vi "Yellow 1 to 2.vi"   [LabVIEW 2019]
uses:
  Global Var.vi
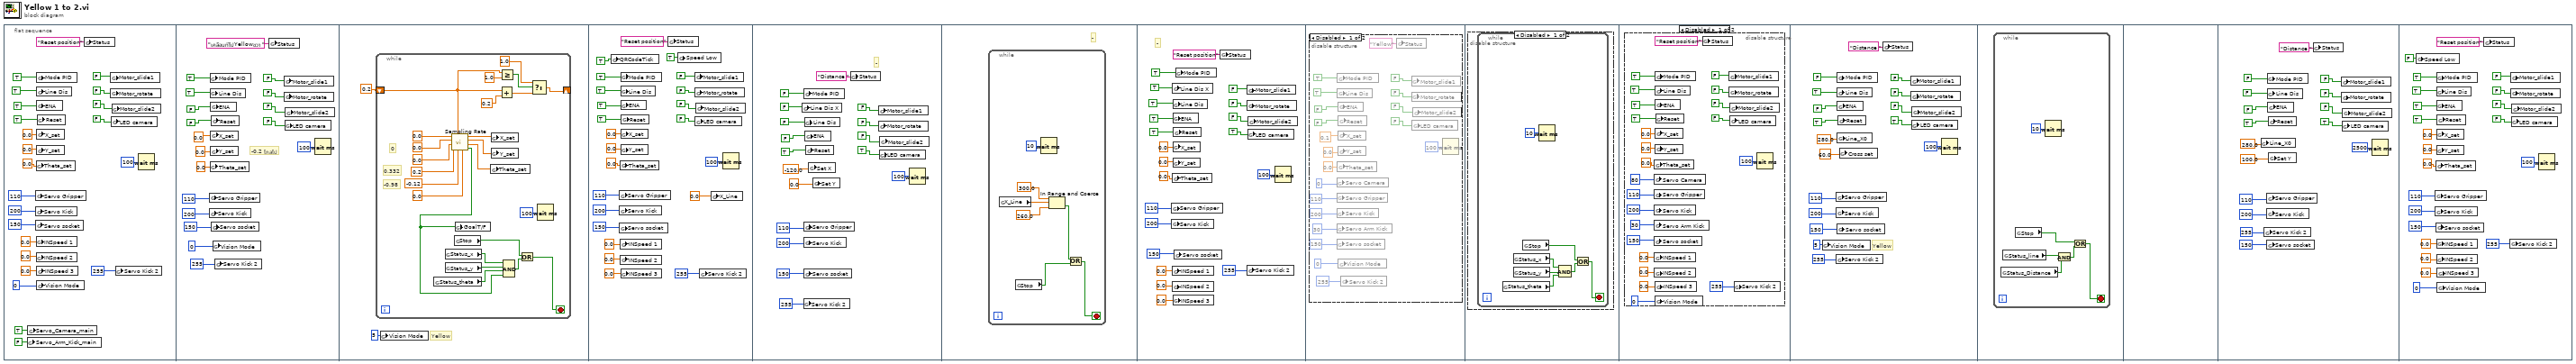
[diagram p0: block diagram]
diagram:
  n1 = flat-sequence {
    frame #0 {
      n2 = global write "Global Var.vi" "Servo_Arm_Kick_main"(FALSE ("Mode PID")) -> ()
      n3 = global write "Global Var.vi" "Servo_Camera_main"(TRUE ("Mode PID")) -> ()
      n4 = global write "Global Var.vi" "Servo Gripper"(u8 110 ("Servo Camera")) -> ()
      n5 = global write "Global Var.vi" "Servo Kick"(u8 200 ("Servo Camera")) -> ()
      n6 = global write "Global Var.vi" "Servo socket"(u8 150 ("Servo Camera")) -> ()
      n7 = global write "Global Var.vi" "Theta_set"(0.0 ("Theta_set")) -> ()
      n8 = global write "Global Var.vi" "INSpeed 1"(0.0 ("X_set")) -> ()
      n9 = global write "Global Var.vi" "INSpeed 2"(0.0 ("Y_set")) -> ()
      n10 = global write "Global Var.vi" "Mode PID"(TRUE ("Mode PID")) -> ()
      n11 = global write "Global Var.vi" "Line Dis"(TRUE ("Mode PID")) -> ()
      n12 = global write "Global Var.vi" "ENA"(TRUE ("ENA")) -> ()
      n13 = global write "Global Var.vi" "X_set"(0.0 ("X_set")) -> ()
      n14 = global write "Global Var.vi" "Y_set"(0.0 ("Y_set")) -> ()
      n15 = global write "Global Var.vi" "INSpeed 3"(0.0 ("Theta_set")) -> ()
      n16 = global write "Global Var.vi" "Vision Mode"(i16 0 ("Vision Mode")) -> ()
      n17 = global write "Global Var.vi" "Reset"(TRUE ("ENA")) -> ()
      n18 = global write "Global Var.vi" "Status"("Reset position" ("Status")) -> ()
      n19 = global write "Global Var.vi" "Motor_slide1"(FALSE ("Mode PID")) -> ()
      n20 = global write "Global Var.vi" "Motor_rotate"(FALSE ("ENA")) -> ()
      n21 = global write "Global Var.vi" "LED camera"(FALSE ("LED camera")) -> ()
      n22 = global write "Global Var.vi" "Motor_slide2"(FALSE ("ENA")) -> ()
      n23 = global write "Global Var.vi" "Servo Kick 2"(u8 255 ("Servo Camera")) -> ()
      n24 = Wait (ms)(milliseconds to wait=u32 100) -> ()  [unwired: 1 out]
    }
    frame #1 {
      # "-0.2 ไกลไป"
      n25 = global write "Global Var.vi" "Servo Gripper"(u8 110 ("Servo Camera")) -> ()
      n26 = global write "Global Var.vi" "Servo Kick"(u8 200 ("Servo Camera")) -> ()
      n27 = global write "Global Var.vi" "Mode PID"(TRUE ("Mode PID")) -> ()
      n28 = global write "Global Var.vi" "Line Dis"(TRUE ("Mode PID")) -> ()
      n29 = global write "Global Var.vi" "Theta_set"(0.0 ("Theta_set")) -> ()
      n30 = global write "Global Var.vi" "ENA"(FALSE ("ENA")) -> ()
      n31 = global write "Global Var.vi" "X_set"(0.0 ("X_set")) -> ()
      n32 = global write "Global Var.vi" "Y_set"(0.0 ("Y_set")) -> ()
      n33 = global write "Global Var.vi" "Reset"(FALSE ("ENA")) -> ()
      n34 = global write "Global Var.vi" "Servo socket"(u8 150 ("Servo Camera")) -> ()
      n35 = global write "Global Var.vi" "Vision Mode"(i16 0 ("Vision Mode")) -> ()
      n36 = global write "Global Var.vi" "Servo Kick 2"(u8 255 ("Servo Camera")) -> ()
      n37 = global write "Global Var.vi" "Status"("เคลื่อนที่ไปYellowขวา " ("Status")) -> ()
      n38 = global write "Global Var.vi" "Motor_slide1"(FALSE ("Mode PID")) -> ()
      n39 = global write "Global Var.vi" "Motor_rotate"(FALSE ("ENA")) -> ()
      n40 = global write "Global Var.vi" "LED camera"(FALSE ("LED camera")) -> ()
      n41 = global write "Global Var.vi" "Motor_slide2"(FALSE ("ENA")) -> ()
      n42 = Wait (ms)(milliseconds to wait=u32 100) -> ()  [unwired: 1 out]
    }
    frame #2 {
      # "Yellow"
      n43 = while {
        shift-right: [w46] -> _
        shift-left: 0.2 -> [w44]
        stop <- w63 stop-if-true
        # "-0.98"
        # "0"
        # "0.332"
        n44 = global read "Global Var.vi" "Status_theta"() -> (w65:bool)
        n45 = global read "Global Var.vi" "Status_x"() -> (w66:bool)
        n46 = global read "Global Var.vi" "Status_y"() -> (w67:bool)
        n47 = call "Sampling Rate.vi"("input a1"=0.0, "input y1"=-0.12, "T(0-1)"=w44, "input x1"=0.2, "input a0"=0.0, "input y0"=0.0, "input x0"=0.0) -> ("GoalT/F"=w51:bool, "a_output"=w58:dbl, "y_output"=w59:dbl, "x_output"=w60:dbl)  [unwired: 1 in]
        n48 = global read "Global Var.vi" "Stop"() -> (w61:bool)
        n49 = global write "Global Var.vi" "GoalT/F"(w51) -> ()
        n50 = global write "Global Var.vi" "Theta_set"(w58) -> ()
        n51 = global write "Global Var.vi" "X_set"(w60) -> ()
        n52 = global write "Global Var.vi" "Y_set"(w59) -> ()
        n53 = Add(x=w44, y=0.2) -> (x+y=w49:dbl)
        n54 = Greater Or Equal?(x=w44, y=1.0) -> (x >= y?=w48:bool)
        n55 = Compound Arithmetic op=AND(w66, w67, w65, w51) -> (w62:bool)
        n56 = Or(x=w61, y=w62) -> (x .or. y?=w63:bool)
        n57 = Select(t=1.0, s=w48, f=w49) -> (s? t:f=w46:dbl)
        n58 = Wait (ms)(milliseconds to wait=u32 100) -> ()  [unwired: 1 out]
      }
      n59 = global write "Global Var.vi" "Vision Mode"(i16 5 ("Vision Mode")) -> ()
    }
    frame #3 {
      n60 = global write "Global Var.vi" "QRCodeTick"(TRUE ("ENA")) -> ()
      n61 = global write "Global Var.vi" "Servo Gripper"(u8 110 ("Servo Camera")) -> ()
      n62 = global write "Global Var.vi" "Servo Kick"(u8 200 ("Servo Camera")) -> ()
      n63 = global write "Global Var.vi" "Servo socket"(u8 150 ("Servo Camera")) -> ()
      n64 = global write "Global Var.vi" "Theta_set"(0.0 ("Theta_set")) -> ()
      n65 = global write "Global Var.vi" "INSpeed 1"(0.0 ("X_set")) -> ()
      n66 = global write "Global Var.vi" "INSpeed 2"(0.0 ("Y_set")) -> ()
      n67 = global write "Global Var.vi" "Mode PID"(TRUE ("Mode PID")) -> ()
      n68 = global write "Global Var.vi" "Line Dis"(TRUE ("Mode PID")) -> ()
      n69 = global write "Global Var.vi" "ENA"(TRUE ("ENA")) -> ()
      n70 = global write "Global Var.vi" "X_set"(0.0 ("X_set")) -> ()
      n71 = global write "Global Var.vi" "Y_set"(0.0 ("Y_set")) -> ()
      n72 = global write "Global Var.vi" "INSpeed 3"(0.0 ("Theta_set")) -> ()
      n73 = global write "Global Var.vi" "Reset"(TRUE ("ENA")) -> ()
      n74 = global write "Global Var.vi" "Status"("Reset position" ("Status")) -> ()
      n75 = global write "Global Var.vi" "Speed Low"(TRUE ("ENA")) -> ()
      n76 = global write "Global Var.vi" "Motor_slide1"(FALSE ("Mode PID")) -> ()
      n77 = global write "Global Var.vi" "Motor_rotate"(FALSE ("ENA")) -> ()
      n78 = global write "Global Var.vi" "LED camera"(FALSE ("LED camera")) -> ()
      n79 = global write "Global Var.vi" "Motor_slide2"(FALSE ("ENA")) -> ()
      n80 = global write "Global Var.vi" "Servo Kick 2"(u8 255 ("Servo Camera")) -> ()
      n81 = global write "Global Var.vi" "X_Line"(0.0 ("X_set")) -> ()
      n82 = Wait (ms)(milliseconds to wait=u32 100) -> ()  [unwired: 1 out]
    }
    frame #4 {
      # "-"
      n83 = global write "Global Var.vi" "Line Dis X"(FALSE ("Mode PID")) -> ()
      n84 = global write "Global Var.vi" "Servo Kick 2"(u8 255 ("Servo Camera")) -> ()
      n85 = global write "Global Var.vi" "Mode PID"(FALSE ("Mode PID")) -> ()
      n86 = global write "Global Var.vi" "Servo Gripper"(u8 110 ("Servo Camera")) -> ()
      n87 = global write "Global Var.vi" "Servo Kick"(u8 200 ("Servo Camera")) -> ()
      n88 = global write "Global Var.vi" "Servo socket"(u8 150 ("Servo Camera")) -> ()
      n89 = global write "Global Var.vi" "Line Dis"(FALSE ("Mode PID")) -> ()
      n90 = global write "Global Var.vi" "ENA"(FALSE ("ENA")) -> ()
      n91 = global write "Global Var.vi" "Reset"(TRUE ("ENA")) -> ()
      n92 = global write "Global Var.vi" "Set X"(-120.0 ("Y_set")) -> ()
      n93 = global write "Global Var.vi" "Set Y"(0.0 ("Y_set")) -> ()
      n94 = global write "Global Var.vi" "Status"("Distance " ("Status")) -> ()
      n95 = global write "Global Var.vi" "Motor_slide1"(FALSE ("Mode PID")) -> ()
      n96 = global write "Global Var.vi" "Motor_rotate"(FALSE ("ENA")) -> ()
      n97 = global write "Global Var.vi" "LED camera"(TRUE ("LED camera")) -> ()
      n98 = global write "Global Var.vi" "Motor_slide2"(FALSE ("ENA")) -> ()
      n99 = Wait (ms)(milliseconds to wait=u32 100) -> ()  [unwired: 1 out]
    }
    frame #5 {
      # "-"
      n100 = while {
        stop <- w113 stop-if-true
        n101 = global read "Global Var.vi" "X_Line"() -> (w111:dbl)
        n102 = global read "Global Var.vi" "Stop"() -> (w112:bool)
        n103 = Wait (ms)(milliseconds to wait=u32 10) -> ()  [unwired: 1 out]
        n104 = In Range and Coerce(upper limit=300.0, x=w111, lower limit=260.0) -> (In Range?=w108:bool)  [unwired: 1 out]
        n105 = Or(x=w108, y=w112) -> (x .or. y?=w113:bool)
      }
    }
    frame #6 {
      # "-"
      n106 = global write "Global Var.vi" "Servo Gripper"(u8 110 ("Servo Camera")) -> ()
      n107 = global write "Global Var.vi" "Servo Kick"(u8 200 ("Servo Camera")) -> ()
      n108 = global write "Global Var.vi" "Line Dis X"(TRUE ("Mode PID")) -> ()
      n109 = global write "Global Var.vi" "Theta_set"(0.0 ("Theta_set")) -> ()
      n110 = global write "Global Var.vi" "INSpeed 1"(0.0 ("X_set")) -> ()
      n111 = global write "Global Var.vi" "INSpeed 2"(0.0 ("Y_set")) -> ()
      n112 = global write "Global Var.vi" "Line Dis"(TRUE ("Mode PID")) -> ()
      n113 = global write "Global Var.vi" "ENA"(TRUE ("ENA")) -> ()
      n114 = global write "Global Var.vi" "X_set"(0.0 ("X_set")) -> ()
      n115 = global write "Global Var.vi" "Y_set"(0.0 ("Y_set")) -> ()
      n116 = global write "Global Var.vi" "INSpeed 3"(0.0 ("Theta_set")) -> ()
      n117 = global write "Global Var.vi" "Reset"(TRUE ("ENA")) -> ()
      n118 = global write "Global Var.vi" "Servo socket"(u8 150 ("Servo Camera")) -> ()
      n119 = global write "Global Var.vi" "Mode PID"(TRUE ("Mode PID")) -> ()
      n120 = global write "Global Var.vi" "Status"("Reset position" ("Status")) -> ()
      n121 = global write "Global Var.vi" "Motor_slide1"(FALSE ("Mode PID")) -> ()
      n122 = global write "Global Var.vi" "Motor_rotate"(FALSE ("ENA")) -> ()
      n123 = global write "Global Var.vi" "Servo Kick 2"(u8 255 ("Servo Camera")) -> ()
      n124 = global write "Global Var.vi" "LED camera"(TRUE ("LED camera")) -> ()
      n125 = global write "Global Var.vi" "Motor_slide2"(FALSE ("ENA")) -> ()
      n126 = Wait (ms)(milliseconds to wait=u32 100) -> ()  [unwired: 1 out]
    }
    frame #7 {
      n127 = disable-structure shown="Disabled" {
        frame Disabled {
          n128 = global write "Global Var.vi" "Servo Camera"(u8 0 ("Servo Camera")) -> ()
          n129 = global write "Global Var.vi" "Servo Gripper"(u8 110 ("Servo Camera")) -> ()
          n130 = global write "Global Var.vi" "Servo Kick"(u8 200 ("Servo Camera")) -> ()
          n131 = global write "Global Var.vi" "Servo Arm Kick"(u8 30 ("Servo Camera")) -> ()
          n132 = global write "Global Var.vi" "Servo socket"(u8 150 ("Servo Camera")) -> ()
          n133 = global write "Global Var.vi" "Mode PID"(TRUE ("Mode PID")) -> ()
          n134 = global write "Global Var.vi" "Line Dis"(TRUE ("Mode PID")) -> ()
          n135 = global write "Global Var.vi" "Theta_set"(0.0 ("Theta_set")) -> ()
          n136 = global write "Global Var.vi" "ENA"(FALSE ("ENA")) -> ()
          n137 = global write "Global Var.vi" "X_set"(0.1 ("X_set")) -> ()
          n138 = global write "Global Var.vi" "Y_set"(0.0 ("Y_set")) -> ()
          n139 = global write "Global Var.vi" "Reset"(FALSE ("ENA")) -> ()
          n140 = global write "Global Var.vi" "Vision Mode"(i16 0 ("Vision Mode")) -> ()
          n141 = global write "Global Var.vi" "Servo Kick 2"(u8 255 ("Servo Camera")) -> ()
          n142 = global write "Global Var.vi" "Status"("Yellow" ("Status")) -> ()
          n143 = global write "Global Var.vi" "Motor_slide1"(FALSE ("Mode PID")) -> ()
          n144 = global write "Global Var.vi" "Motor_rotate"(FALSE ("ENA")) -> ()
          n145 = global write "Global Var.vi" "LED camera"(FALSE ("LED camera")) -> ()
          n146 = global write "Global Var.vi" "Motor_slide2"(FALSE ("ENA")) -> ()
          n147 = Wait (ms)(milliseconds to wait=u32 100) -> ()  [unwired: 1 out]
        }
        frame Enabled {
        }
      }
    }
    frame #8 {
      n148 = disable-structure shown="Disabled" {
        frame Disabled {
          n149 = while {
            stop <- w158 stop-if-true
            n150 = global read "Global Var.vi" "Status_theta"() -> (w160:bool)
            n151 = global read "Global Var.vi" "Status_x"() -> (w161:bool)
            n152 = global read "Global Var.vi" "Status_y"() -> (w162:bool)
            n153 = global read "Global Var.vi" "Stop"() -> (w156:bool)
            n154 = Wait (ms)(milliseconds to wait=u32 10) -> ()  [unwired: 1 out]
            n155 = Compound Arithmetic op=AND(w161, w162, w160) -> (w157:bool)
            n156 = Or(x=w156, y=w157) -> (x .or. y?=w158:bool)
          }
        }
        frame Enabled {
        }
      }
    }
    frame #9 {
      n157 = disable-structure shown="Disabled" {
        frame Disabled {
          n158 = global write "Global Var.vi" "Servo Camera"(u8 80 ("Servo Camera")) -> ()
          n159 = global write "Global Var.vi" "Servo Gripper"(u8 110 ("Servo Camera")) -> ()
          n160 = global write "Global Var.vi" "Servo Kick"(u8 200 ("Servo Camera")) -> ()
          n161 = global write "Global Var.vi" "Servo Arm Kick"(u8 30 ("Servo Camera")) -> ()
          n162 = global write "Global Var.vi" "Servo socket"(u8 150 ("Servo Camera")) -> ()
          n163 = global write "Global Var.vi" "Theta_set"(0.0 ("Theta_set")) -> ()
          n164 = global write "Global Var.vi" "INSpeed 1"(0.0 ("X_set")) -> ()
          n165 = global write "Global Var.vi" "INSpeed 2"(0.0 ("Y_set")) -> ()
          n166 = global write "Global Var.vi" "Mode PID"(TRUE ("Mode PID")) -> ()
          n167 = global write "Global Var.vi" "Line Dis"(TRUE ("Mode PID")) -> ()
          n168 = global write "Global Var.vi" "ENA"(TRUE ("ENA")) -> ()
          n169 = global write "Global Var.vi" "X_set"(0.0 ("X_set")) -> ()
          n170 = global write "Global Var.vi" "Y_set"(0.0 ("Y_set")) -> ()
          n171 = global write "Global Var.vi" "INSpeed 3"(0.0 ("Theta_set")) -> ()
          n172 = global write "Global Var.vi" "Vision Mode"(i16 0 ("Vision Mode")) -> ()
          n173 = global write "Global Var.vi" "Reset"(TRUE ("ENA")) -> ()
          n174 = global write "Global Var.vi" "Status"("Reset position" ("Status")) -> ()
          n175 = global write "Global Var.vi" "Motor_slide1"(FALSE ("Mode PID")) -> ()
          n176 = global write "Global Var.vi" "Motor_rotate"(FALSE ("ENA")) -> ()
          n177 = global write "Global Var.vi" "LED camera"(FALSE ("LED camera")) -> ()
          n178 = global write "Global Var.vi" "Motor_slide2"(FALSE ("ENA")) -> ()
          n179 = global write "Global Var.vi" "Servo Kick 2"(u8 255 ("Servo Camera")) -> ()
          n180 = Wait (ms)(milliseconds to wait=u32 100) -> ()  [unwired: 1 out]
        }
        frame Enabled {
        }
      }
    }
    frame #10 {
      # "Yellow"
      n181 = global write "Global Var.vi" "Vision Mode"(i16 5 ("Vision Mode")) -> ()
      n182 = global write "Global Var.vi" "Servo Gripper"(u8 110 ("Servo Camera")) -> ()
      n183 = global write "Global Var.vi" "Servo Kick"(u8 200 ("Servo Camera")) -> ()
      n184 = global write "Global Var.vi" "Servo Kick 2"(u8 255 ("Servo Camera")) -> ()
      n185 = global write "Global Var.vi" "Mode PID"(FALSE ("Mode PID")) -> ()
      n186 = global write "Global Var.vi" "Line Dis"(TRUE ("Mode PID")) -> ()
      n187 = global write "Global Var.vi" "Servo socket"(u8 150 ("Servo Camera")) -> ()
      n188 = global write "Global Var.vi" "ENA"(FALSE ("ENA")) -> ()
      n189 = global write "Global Var.vi" "Line_X0"(280.0 ("Y_set")) -> ()
      n190 = global write "Global Var.vi" "Reset"(TRUE ("ENA")) -> ()
      n191 = global write "Global Var.vi" "Cross set"(60.0 ("Y_set")) -> ()
      n192 = global write "Global Var.vi" "Status"("Distance " ("Status")) -> ()
      n193 = global write "Global Var.vi" "Motor_slide1"(FALSE ("Mode PID")) -> ()
      n194 = global write "Global Var.vi" "Motor_rotate"(FALSE ("ENA")) -> ()
      n195 = global write "Global Var.vi" "LED camera"(TRUE ("LED camera")) -> ()
      n196 = global write "Global Var.vi" "Motor_slide2"(FALSE ("ENA")) -> ()
      n197 = Wait (ms)(milliseconds to wait=u32 100) -> ()  [unwired: 1 out]
    }
    frame #11 {
      n198 = while {
        stop <- w207 stop-if-true
        n199 = global read "Global Var.vi" "Status_Distance"() -> (w203:bool)
        n200 = global read "Global Var.vi" "Status_line"() -> (w204:bool)
        n201 = global read "Global Var.vi" "Stop"() -> (w206:bool)
        n202 = Wait (ms)(milliseconds to wait=u32 10) -> ()  [unwired: 1 out]
        n203 = And(x=w204, y=w203) -> (x .and. y?=w205:bool)
        n204 = Or(x=w206, y=w205) -> (x .or. y?=w207:bool)
      }
    }
    frame #12 {
    }
    frame #13 {
      n205 = global write "Global Var.vi" "Line_X0"(280.0 ("Y_set")) -> ()
      n206 = global write "Global Var.vi" "Servo Kick 2"(u8 255 ("Servo Camera")) -> ()
      n207 = global write "Global Var.vi" "Servo Gripper"(u8 110 ("Servo Camera")) -> ()
      n208 = global write "Global Var.vi" "Servo Kick"(u8 200 ("Servo Camera")) -> ()
      n209 = global write "Global Var.vi" "Servo socket"(u8 150 ("Servo Camera")) -> ()
      n210 = global write "Global Var.vi" "Mode PID"(FALSE ("Mode PID")) -> ()
      n211 = global write "Global Var.vi" "Line Dis"(FALSE ("Mode PID")) -> ()
      n212 = global write "Global Var.vi" "ENA"(FALSE ("ENA")) -> ()
      n213 = global write "Global Var.vi" "Reset"(TRUE ("ENA")) -> ()
      n214 = global write "Global Var.vi" "Set Y"(100.0 ("Y_set")) -> ()
      n215 = global write "Global Var.vi" "Status"("Distance " ("Status")) -> ()
      n216 = global write "Global Var.vi" "Motor_slide1"(FALSE ("Mode PID")) -> ()
      n217 = global write "Global Var.vi" "Motor_rotate"(FALSE ("ENA")) -> ()
      n218 = global write "Global Var.vi" "LED camera"(TRUE ("LED camera")) -> ()
      n219 = global write "Global Var.vi" "Motor_slide2"(FALSE ("ENA")) -> ()
      n220 = Wait (ms)(milliseconds to wait=u32 2500) -> ()  [unwired: 1 out]
    }
    frame #14 {
      n221 = global write "Global Var.vi" "Speed Low"(FALSE ("ENA")) -> ()
      n222 = global write "Global Var.vi" "Servo Gripper"(u8 110 ("Servo Camera")) -> ()
      n223 = global write "Global Var.vi" "Servo Kick"(u8 200 ("Servo Camera")) -> ()
      n224 = global write "Global Var.vi" "Theta_set"(0.0 ("Theta_set")) -> ()
      n225 = global write "Global Var.vi" "Servo socket"(u8 150 ("Servo Camera")) -> ()
      n226 = global write "Global Var.vi" "Mode PID"(TRUE ("Mode PID")) -> ()
      n227 = global write "Global Var.vi" "Line Dis"(TRUE ("Mode PID")) -> ()
      n228 = global write "Global Var.vi" "ENA"(TRUE ("ENA")) -> ()
      n229 = global write "Global Var.vi" "X_set"(0.0 ("X_set")) -> ()
      n230 = global write "Global Var.vi" "Y_set"(0.0 ("Y_set")) -> ()
      n231 = global write "Global Var.vi" "INSpeed 1"(0.0 ("X_set")) -> ()
      n232 = global write "Global Var.vi" "INSpeed 2"(0.0 ("Y_set")) -> ()
      n233 = global write "Global Var.vi" "Reset"(TRUE ("ENA")) -> ()
      n234 = global write "Global Var.vi" "INSpeed 3"(0.0 ("Theta_set")) -> ()
      n235 = global write "Global Var.vi" "Vision Mode"(i16 0 ("Vision Mode")) -> ()
      n236 = global write "Global Var.vi" "Status"("Reset position" ("Status")) -> ()
      n237 = global write "Global Var.vi" "Servo Kick 2"(u8 255 ("Servo Camera")) -> ()
      n238 = global write "Global Var.vi" "Motor_slide1"(FALSE ("Mode PID")) -> ()
      n239 = global write "Global Var.vi" "Motor_rotate"(FALSE ("ENA")) -> ()
      n240 = global write "Global Var.vi" "LED camera"(FALSE ("LED camera")) -> ()
      n241 = global write "Global Var.vi" "Motor_slide2"(FALSE ("ENA")) -> ()
      n242 = Wait (ms)(milliseconds to wait=u32 100) -> ()  [unwired: 1 out]
    }
  }
